vi "getPressure.vi"(3 "error in":errorcluster, 4 "AIN Range":u16(ring) items=["LJ_rgBIP10V", "LJ_rgBIP1V", "LJ_rgBIPP1V", "LJ_rgBIPP01V"], 5 "+Channel":u16, 6 "Handle In":i32) -> (0 "error out":errorcluster, 1 "Pressure Reading":dbl, 2 "Voltage Reading":dbl)   [LabVIEW 2021]
panel:
  # "inputs"
  # "outputs"
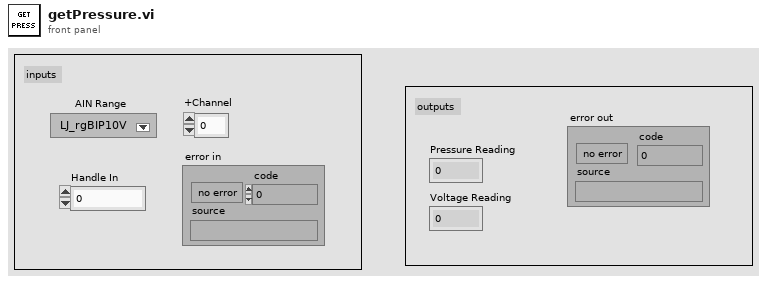
[diagram p1: front panel]
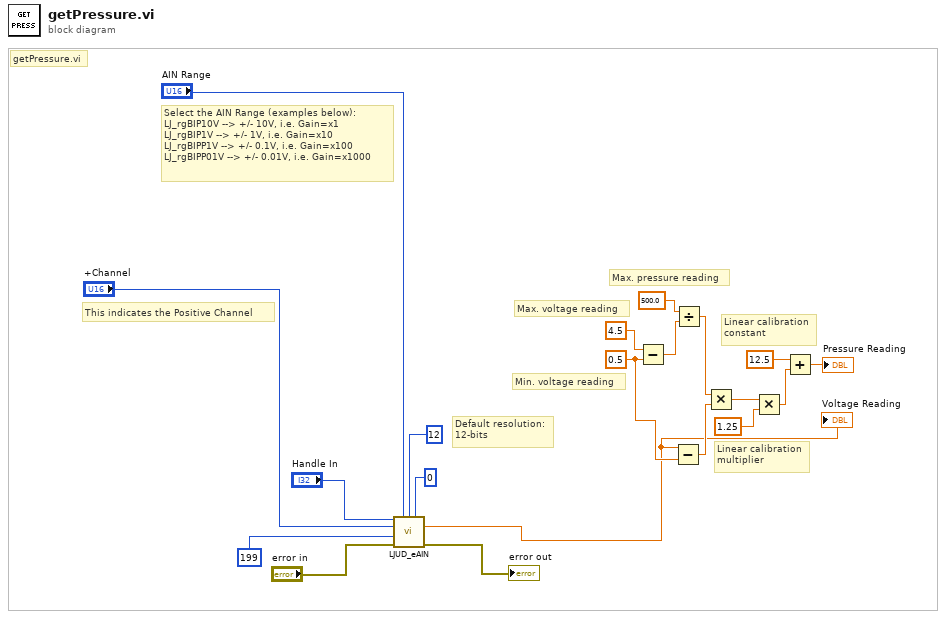
[diagram p0: block diagram]
diagram:
  w15 = 0.5 ("y")
  # "Linear calibration\nconstant"
  # "Linear calibration\nmultiplier"
  # "Min. voltage reading"
  # "Max. voltage reading"
  # "Max. pressure reading"
  # "getPressure.vi"
  # "This indicates the Positive Channel"
  # "Default resolution:\n12-bits"
  # "Select the AIN Range (examples below):\nLJ_rgBIP10V --> +/- 10V, i.e. Gain=x1\nLJ_rgBIP1V --> +/- 1V, i.e. Gain=x10\nLJ_rgBIPP1V --> +/- 0.1V, i.e. Gain=x100\nLJ_rgBIPP01V --> +/- 0.01V, i.e. Gain=x1000"
  n1 = call <vilib>:"LJUD_eAIN.vi"("Handle In"="Handle In", "Range"="AIN Range", "Resolution"=12, "Settling"=0, "ChannelP"="+Channel", "ChannelN"=199, "error in"="error in") -> ("Voltage"=w2:dbl, "error out"=→"error out":errorcluster)  [unwired: 6 in, 1 out]
  "Voltage Reading" <- w2
  n2 = Subtract(x=4.5, y=w15) -> (x-y=w18:dbl)
  n3 = Subtract(x=w2, y=w15) -> (x-y=w16:dbl)
  n4 = Divide(x=500.0 ("y"), y=w18) -> (x/y=w17:dbl)
  n5 = Multiply(x=w17, y=w16) -> (x*y=w14:dbl)
  n6 = Multiply(x=w14, y=1.25) -> (x*y=w11:dbl)
  n7 = Add(x=12.5, y=w11) -> (x+y=→"Pressure Reading":dbl)
